vi "set plugin type.vi"(8 "error in (no error)":errorcluster, 9 "plugin type":string, 10 "id":string, 11 "DSFConfiguration in":refnum<class "DSFConfiguration.lvclass">) -> (0 "error out":errorcluster, 3 "DSFConfiguration out":refnum<class "DSFConfiguration.lvclass">)   [LabVIEW 2017, in "DSFConfiguration.lvclass"]
uses:
  DSFConfiguration.lvclass
  DSFConfiguration.lvclass/DSFConfiguration.ctl
  DSFPlugin/DSFPlugin.lvclass/DSFPlugin.ctl
  DSFPlugin/DSFPlugin.lvclass
  C:/github/data-sharing-framework/Source/Configuration API/Classes/IDable/IDable.lvclass
  ID API/ID API.lvclass
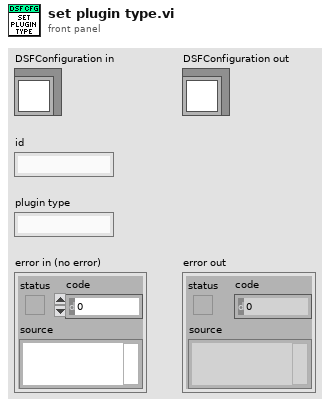
[diagram p1: front panel]
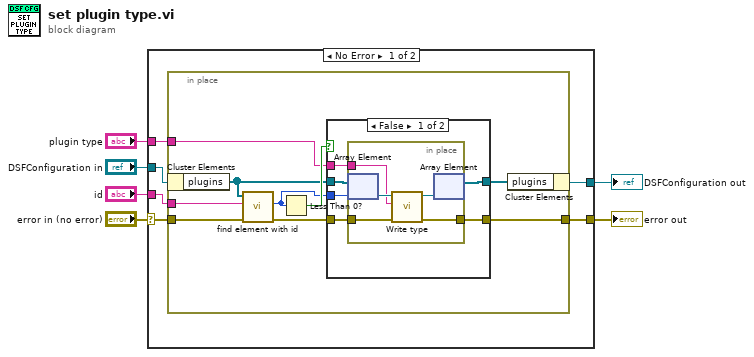
[diagram p0: block diagram]
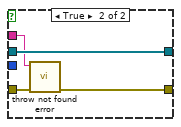
[diagram p2: hidden frame]
diagram:
  n1 = case shown="No Error" "error in (no error)" {
    selector: "error in (no error)" -> [w10 w38]
    tunnel: [w8 w38] -> w5
    tunnel: [w9 w37] -> w3
    tunnel: "DSFConfiguration in" -> [w12 w37]
    tunnel: "id" -> [w11 _]
    tunnel: "plugin type" -> [w7 _]
    frame No Error {
      n2 = in-place {
        in-place-border: w11 -> [w21]
        in-place-border: w10 -> [w20]
        in-place-border: [w17] -> w8
        in-place-border: w7 -> [w14]
        n3 = in-place-cluster #1(w12) -> ("plugins"=w16:refnum<class "DSFPlugin.lvclass">[])
        n4 = call "find element with id.vi"("error in (no error)"=w20, "id"=w21, "IDable Array in"=w16) -> ("error out"=w18:errorcluster, "index"=w15:i32)  [unwired: 7 in]
        n5 = Less Than 0?(x=w15) -> (x < 0?=w19:bool)
        n6 = case shown="False" w19 {
          tunnel: w18 -> [w24 w33]
          tunnel: [w23 w36] -> w17
          tunnel: w16 -> [w27 w35]
          tunnel: w15 -> [w26 _]
          tunnel: w14 -> [w25 w34]
          tunnel: [w22 w35] -> w13
          frame False {
            n7 = in-place {
              in-place-border: w25 -> [w28]
              in-place-border: w24 -> [w32]
              in-place-border: [w31] -> w23
              n8 = in-place-array #2(w27, w26) -> (w30:refnum<class "DSFPlugin.lvclass">)
              n9 = call "Write type.vi"("error in (no error)"=w32, "type"=w28, "DSFPlugin in"=w30) -> ("error out"=w31:errorcluster, "DSFPlugin out"=w29:refnum<class "DSFPlugin.lvclass">)  [unwired: 7 in]
              n10 = in-place-array #2(w29) -> (w22:refnum<class "DSFPlugin.lvclass">[])  [unwired: 1 out]
            }
          }
          frame True {
            n11 = call "throw not found error.vi"("error in (no error)"=w33, "id"=w34) -> ("error out"=w36:errorcluster)  [unwired: 9 in]
          }
        }
        n12 = in-place-cluster #1("plugins"=w13) -> (w9:refnum<class "DSFConfiguration.lvclass">)
      }
    }
    frame Error {
    }
  }
  "error out" <- w5
  "DSFConfiguration out" <- w3
